vi "Discover_PNA.vi"(8 "error in":errorcluster {"code" format="%.0x"}, 11 "Session In":refnum<visa-resource-name>="TCPIP0::10.0.1.24::inst0::INSTR") -> (0 "error out":errorcluster {"code" format="%.0x"}, 2 "Success?(t)":bool, 3 "Session Out":refnum<visa-resource-name>)   [LabVIEW 2018]
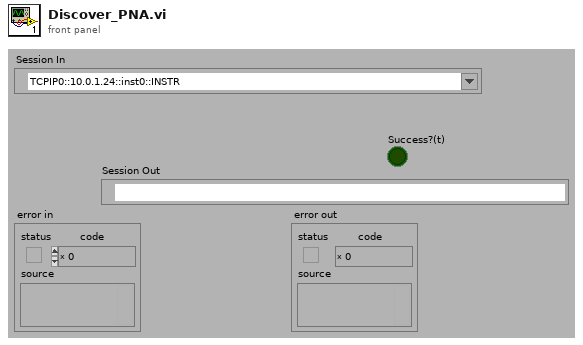
[diagram p1: front panel]
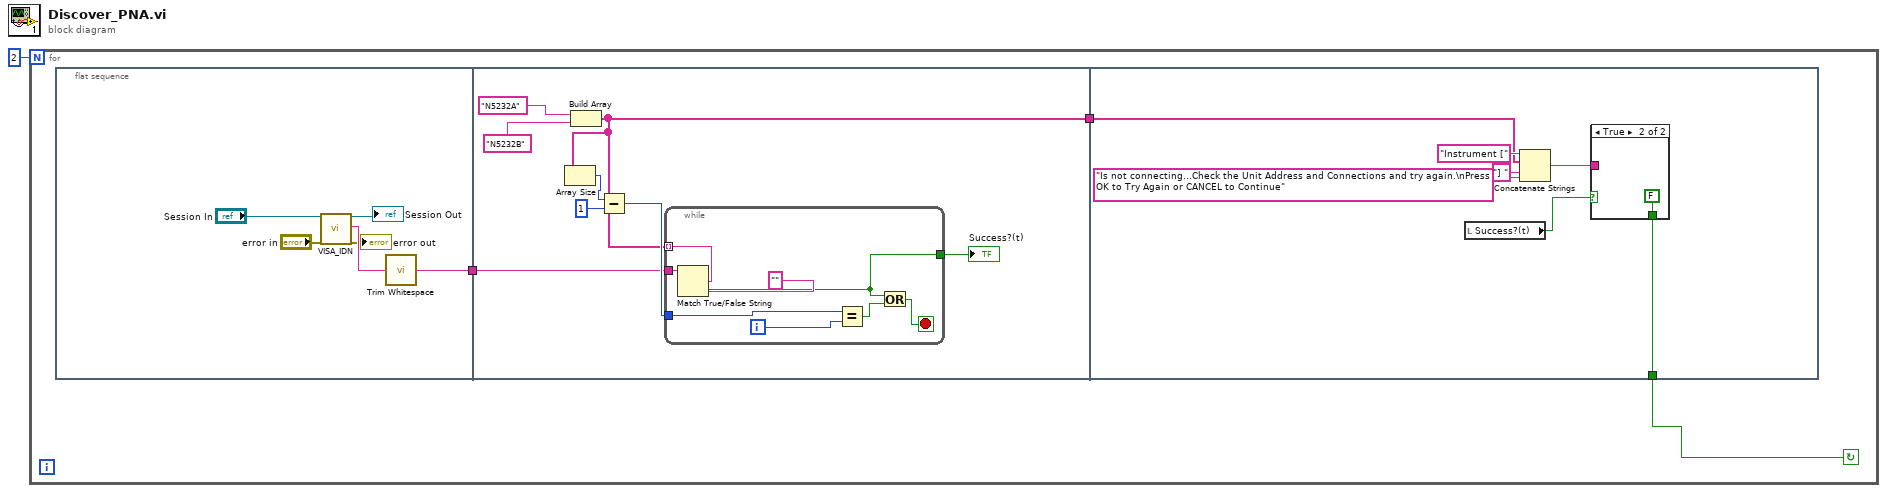
[diagram p0: block diagram]
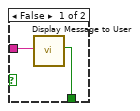
[diagram p2: hidden frame]
diagram:
  n1 = for {
    N: 2 -> [_]
    stop <- w2 continue-if-true
    n2 = flat-sequence {
      tunnel: [w7] -> w4
      tunnel: w4 -> [w14]
      tunnel: [w13] -> w3
      tunnel: w3 -> [w32]
      tunnel: [w27] -> w2
      frame #0 {
        n3 = call "VISA_IDN.vi"("Session In"="Session In", "error in"="error in") -> ("Session Out"=→"Session Out":refnum<visa-resource-name>, "Model"=w10:string, "error out"=→"error out":errorcluster)  [unwired: 11 in, 4 out]
        n4 = call <vilib>:"Trim Whitespace.vi"("string"=w10) -> ("trimmed string"=w7:string)  [unwired: 1 in]
      }
      frame #1 {
        n5 = Build Array("N5232A" ("element"), "N5232B" ("true string")) -> (w13:string[])
        n6 = Array Size(array=w13) -> (size(s)=w17:i32)
        n7 = Subtract(x=w17, y=1) -> (x-y=w15:i32)
        n8 = while {
          tunnel: w13 -> [w25] mode=indexing
          tunnel: w14 -> [w24]
          tunnel: [w23] -> w18
          tunnel: w15 -> [w19]
          i -> [w20]
          stop <- w22 stop-if-true
          n9 = Match True/False String(2:"" ("false string"), 3:w25, 4:w24) -> (0:w23:bool)  [unwired: 1 out]
          n10 = Equal?(x=w19, y=w20) -> (x = y?=w21:bool)
          n11 = Or(x=w23, y=w21) -> (x .or. y?=w22:bool)
        }
        "Success?(t)" <- w18
      }
      frame #2 {
        n12 = local read "Success?(t)"() -> (w28:bool)
        n13 = Concatenate Strings("Instrument [" ("string"), w32, "] " ("string"), "Is not connecting...Check the Unit Address and Connections and try again.\nPress OK to Try Again or CANCEL to Continue" ("string")) -> (w29:string)
        n14 = case shown="True" w28 {
          tunnel: w29 -> [w35 _]
          tunnel: [w34 FALSE ("OK")] -> w27
          frame False {
            n15 = call "Display Message to User"("Message"=w35) -> ("OK"=w34:bool)  [unwired: 9 in, 1 out]
          }
          frame True {
          }
        }
      }
    }
  }
